vi "Disconnect Everything from Typedef.vi"(6 "Variant in":variant, 7 "Shift Pressed?":bool, 8 "error in (no error)":errorcluster, 10 "QD Combo Box Ref":refnum<vi>, 11 "QD Launch VI Ref":refnum<vi>) -> (0 "error out":errorcluster, 4 "Variant out":variant)   [LabVIEW 2017]
doc: "Disconnects all controls (on front panel) or constants (on block diagram) from their source type definition. If [Shift] is also pressed, disconnects all controls/constants within the selection from their source type definitions recursively.\n\nDefault Shortcut - [h]"
uses:
  <vilib>/Utility/traverseref.llb/TRef TravTarget.ctl
  <vilib>/Utility/traverseref.llb/VI Scripting - Traverse.lvlib
panel:
  in  "Undo Name":string="Disconnect from Typedef"
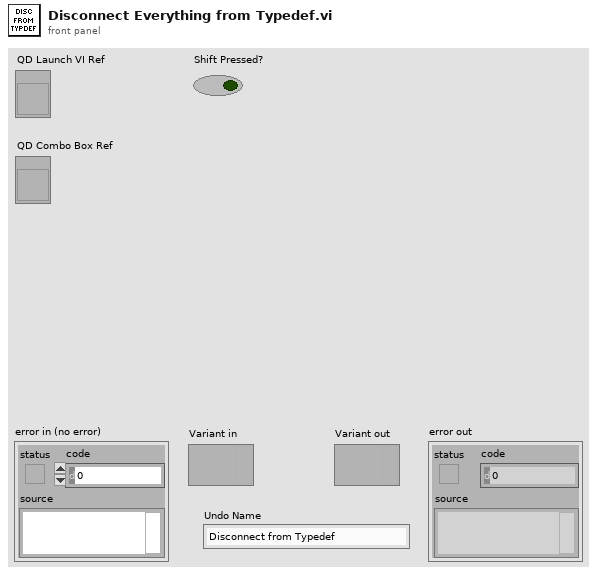
[diagram p1: front panel]
types:
  T1 = typedef "TRef TravTarget.ctl" = enum16{"FP", "BD", "Other"}
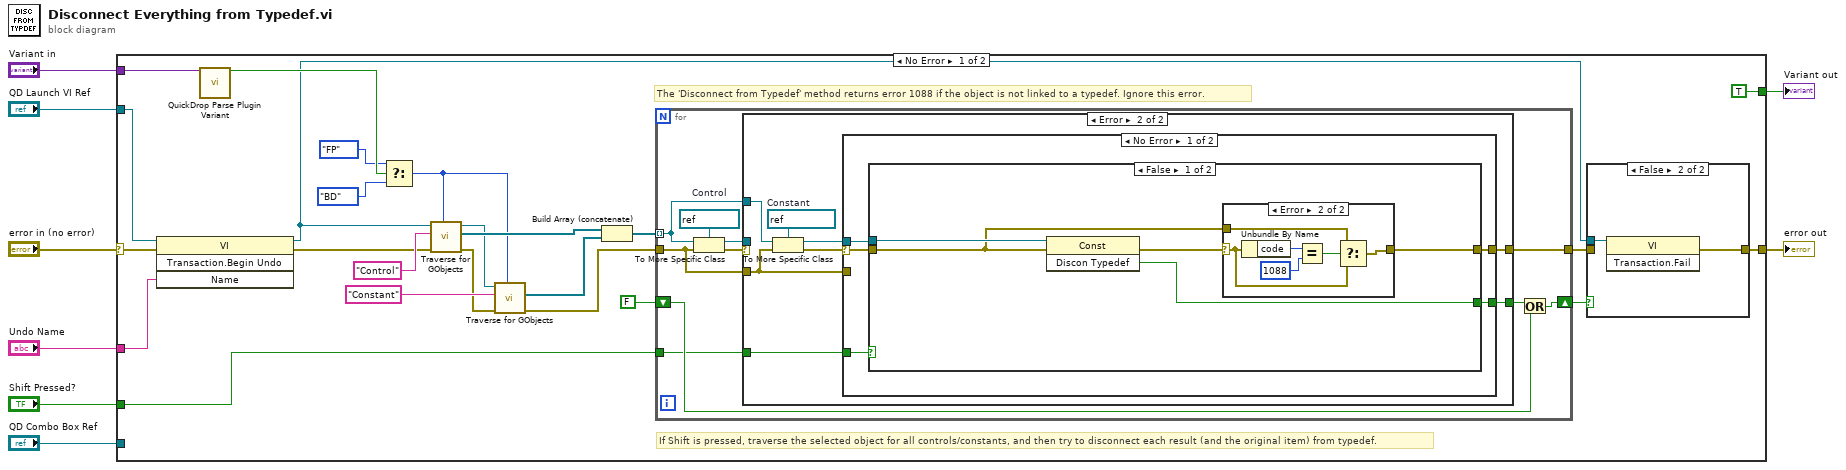
[diagram p0: block diagram]
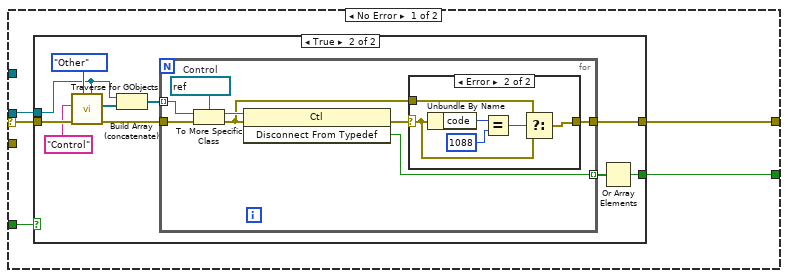
[diagram p2: hidden frame]
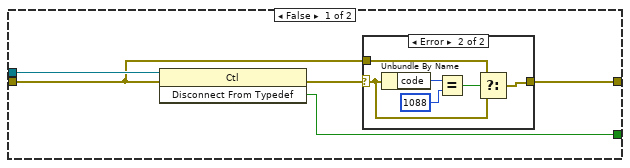
[diagram p3: hidden frame]
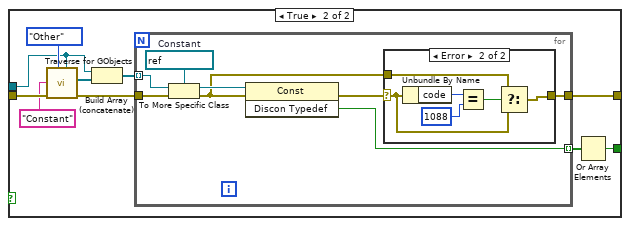
[diagram p7: hidden frame]
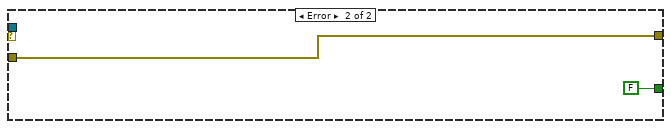
[diagram p9: hidden frame]
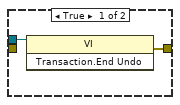
[diagram p10: hidden frame]
diagram:
  n1 = case shown="No Error" "error in (no error)" {
    selector: "error in (no error)" -> [w31 w141]
    tunnel: [w27 w141] -> w7
    tunnel: "QD Launch VI Ref" -> [w30 _]
    tunnel: "Shift Pressed?" -> [w24 _]
    tunnel: "QD Combo Box Ref" -> [_ _]
    tunnel: "Variant in" -> [w32 _]
    tunnel: "Undo Name" -> [w29 _]
    tunnel: [TRUE _] -> w1
    frame No Error {
      # "If Shift is pressed, traverse the selected object for all controls/constants, and then try to disconnect each result (and the original item) from typedef."
      # "The 'Disconnect from Typedef' method returns error 1088 if the object is not linked to a typedef. Ignore this error."
      n2 = invoke class="VI" method="Transaction.Begin Undo"(reference=w30, error in=w31, "Name"=w29) -> (reference out=w17:refnum<vi>, error out=w15:errorcluster)  [unwired: 1 in, 2 out]
      n3 = call <vilib>:"QuickDrop Parse Plugin Variant.vi"("QDKS Variant in"=w32) -> ("QD Launch VI Panel?"=w21:bool)  [unwired: 12 in, 2 out]
      n4 = Select(t=TRef_TravTarget."FP" ("Traverse Target"), s=w21, f=TRef_TravTarget."BD" ("Traverse Target")) -> (s? t:f=w12:T1)
      n5 = call <vilib>:"Traverse for GObjects.vi"("Traverse Target"=w12, "error in (no error)"=w15, "Class Name"="Control", "VI Refnum"=w17) -> ("error out"=w11:errorcluster, "References"=w18:refnum<vi>[], "dup VI Refnum"=w10:refnum<vi>)  [unwired: 4 in, 1 out]
      n6 = call <vilib>:"Traverse for GObjects.vi"("Traverse Target"=w12, "error in (no error)"=w11, "Class Name"="Constant", "VI Refnum"=w10) -> ("error out"=w9:errorcluster, "References"=w13:refnum<vi>[])  [unwired: 4 in, 2 out]
      n7 = Build Array (concatenate)(w18, w13) -> (w14:refnum<vi>[])
      n8 = for {
        shift-right: [w42] -> w25
        shift-left: FALSE -> [w40]
        tunnel: w14 -> [w33] mode=indexing
        tunnel: w9 -> [w34]
        tunnel: [w36] -> w23
        tunnel: w24 -> [w35]
        w41 = refnum<vi> refnum  # Control
        n9 = To More Specific Class(target class=w41, reference=w33, error in=w34) -> (specific class reference=w38:refnum<vi>, error out=w39:errorcluster)
        n10 = case shown="Error" w39 {
          selector: w39 -> [w47 _]
          tunnel: w38 -> [w46 _]
          tunnel: [w45 w86] -> w37
          tunnel: [w44 w88] -> w36
          tunnel: w35 -> [w43 w85]
          tunnel: w34 -> [_ w87]
          tunnel: w33 -> [_ w92]
          frame No Error {
            n11 = case shown="True" w43 {
              tunnel: w47 -> [w49 w67]
              tunnel: w46 -> [w52 w62]
              tunnel: [w51 w60] -> w45
              tunnel: [w48 w68] -> w44
              frame False {
                n12 = invoke class="Ctl" method="Disconnect From Typedef"(reference=w52, error in=w49) -> (error out=w50:errorcluster, "Discon Typedef"=w51:bool)  [unwired: 1 in, 1 out]
                n13 = case shown="Error" w50 {
                  selector: w50 -> [w53 w56]
                  tunnel: [w53 w55] -> w48
                  tunnel: w49 -> [_ w54]
                  frame No Error {
                  }
                  frame Error {
                    n14 = Unbundle By Name(w56) -> ("code"=w59:i32)
                    n15 = Equal?(x=w59, y=1088) -> (x = y?=w57:bool)
                    n16 = Select(t=w54, s=w57, f=w56) -> (s? t:f=w55:errorcluster)
                  }
                }
              }
              frame True {
                n17 = call <vilib>:"Traverse for GObjects.vi"("Other Refnum"=w62, "Traverse Target"=TRef_TravTarget."Other", "error in (no error)"=w67, "Class Name"="Control") -> ("error out"=w64:errorcluster, "References"=w63:refnum<vi>[])  [unwired: 4 in, 2 out]
                n18 = Build Array (concatenate)(w62, w63) -> (w61:refnum<vi>[])
                n19 = for {
                  tunnel: [w77] -> w69 mode=indexing
                  tunnel: [w71] -> w68
                  tunnel: w64 -> [w76]
                  tunnel: w61 -> [w75] mode=indexing
                  w74 = refnum<vi> refnum  # Control
                  n20 = To More Specific Class(target class=w74, reference=w75, error in=w76) -> (specific class reference=w73:refnum<vi>, error out=w70:errorcluster)
                  n21 = invoke class="Ctl" method="Disconnect From Typedef"(reference=w73, error in=w70) -> (error out=w72:errorcluster, "Discon Typedef"=w77:bool)  [unwired: 1 in, 1 out]
                  n22 = case shown="Error" w72 {
                    selector: w72 -> [w78 w81]
                    tunnel: [w78 w80] -> w71
                    tunnel: w70 -> [_ w79]
                    frame No Error {
                    }
                    frame Error {
                      n23 = Unbundle By Name(w81) -> ("code"=w84:i32)
                      n24 = Equal?(x=w84, y=1088) -> (x = y?=w82:bool)
                      n25 = Select(t=w79, s=w82, f=w81) -> (s? t:f=w80:errorcluster)
                    }
                  }
                }
                n26 = Or Array Elements(Boolean array=w69) -> (logical OR=w60:bool)
              }
            }
          }
          frame Error {
            w91 = refnum<vi> refnum  # Constant
            n27 = To More Specific Class(target class=w91, reference=w92, error in=w87) -> (specific class reference=w89:refnum<vi>, error out=w90:errorcluster)
            n28 = case shown="No Error" w90 {
              selector: w90 -> [w97 _]
              tunnel: w89 -> [w96 _]
              tunnel: [w94 w136] -> w88
              tunnel: w87 -> [_ w136]
              tunnel: [w93 FALSE] -> w86
              tunnel: w85 -> [w95 _]
              frame No Error {
                n29 = case shown="False" w95 {
                  tunnel: w97 -> [w99 w117]
                  tunnel: w96 -> [w102 w112]
                  tunnel: [w101 w110] -> w93
                  tunnel: [w98 w118] -> w94
                  frame False {
                    n30 = invoke class="Const" method="Discon Typedef"(reference=w102, error in=w99) -> (error out=w100:errorcluster, "Discon Typedef"=w101:bool)  [unwired: 1 in, 1 out]
                    n31 = case shown="Error" w100 {
                      selector: w100 -> [w103 w106]
                      tunnel: [w103 w105] -> w98
                      tunnel: w99 -> [_ w104]
                      frame No Error {
                      }
                      frame Error {
                        n32 = Unbundle By Name(w106) -> ("code"=w109:i32)
                        n33 = Equal?(x=w109, y=1088) -> (x = y?=w107:bool)
                        n34 = Select(t=w104, s=w107, f=w106) -> (s? t:f=w105:errorcluster)
                      }
                    }
                  }
                  frame True {
                    n35 = call <vilib>:"Traverse for GObjects.vi"("Other Refnum"=w112, "Traverse Target"=TRef_TravTarget."Other", "error in (no error)"=w117, "Class Name"="Constant") -> ("error out"=w114:errorcluster, "References"=w113:refnum<vi>[])  [unwired: 4 in, 2 out]
                    n36 = Build Array (concatenate)(w112, w113) -> (w111:refnum<vi>[])
                    n37 = for {
                      tunnel: [w127] -> w119 mode=indexing
                      tunnel: [w121] -> w118
                      tunnel: w114 -> [w126]
                      tunnel: w111 -> [w125] mode=indexing
                      w124 = refnum<vi> refnum  # Constant
                      n38 = To More Specific Class(target class=w124, reference=w125, error in=w126) -> (specific class reference=w123:refnum<vi>, error out=w120:errorcluster)
                      n39 = invoke class="Const" method="Discon Typedef"(reference=w123, error in=w120) -> (error out=w122:errorcluster, "Discon Typedef"=w127:bool)  [unwired: 1 in, 1 out]
                      n40 = case shown="Error" w122 {
                        selector: w122 -> [w128 w131]
                        tunnel: [w128 w130] -> w121
                        tunnel: w120 -> [_ w129]
                        frame No Error {
                        }
                        frame Error {
                          n41 = Unbundle By Name(w131) -> ("code"=w134:i32)
                          n42 = Equal?(x=w134, y=1088) -> (x = y?=w132:bool)
                          n43 = Select(t=w129, s=w132, f=w131) -> (s? t:f=w130:errorcluster)
                        }
                      }
                    }
                    n44 = Or Array Elements(Boolean array=w119) -> (logical OR=w110:bool)
                  }
                }
              }
              frame Error {
              }
            }
          }
        }
        n45 = Or(x=w37, y=w40) -> (x .or. y?=w42:bool)
      }
      n46 = case shown="False" w25 {
        tunnel: w17 -> [w137 w139]
        tunnel: [w138 w140] -> w27
        tunnel: w23 -> [_ _]
        frame True {
          n47 = invoke class="VI" method="Transaction.End Undo"(reference=w137) -> (error out=w138:errorcluster)  [unwired: 2 in, 2 out]
        }
        frame False {
          n48 = invoke class="VI" method="Transaction.Fail"(reference=w139) -> (error out=w140:errorcluster)  [unwired: 2 in, 2 out]
        }
      }
    }
    frame Error {
    }
  }
  "error out" <- w7
  "Variant out" <- w1
